vi "calcul.vi"(9 "In":dbl[](array[numeric]), 10 "Label (y)":dbl[](array[numeric]), 11 "Data (allx)":dbl[][](array[numeric])) -> (1 "PVAL":dbl[](array[numeric]), 3 "B":dbl[](array[numeric]))   [LabVIEW 2014]
uses:
  <vilib>/Analysis/Matrix/Datatypes/RealMatrix.ctl
  <vilib>/Analysis/baseanly.llb/Mean (DBL).vi
  <vilib>/Analysis/_algsub.llb/Real Vector Norm.vi
  <vilib>/Analysis/7linalg.llb/Real QR Decomposition.vi
  <vilib>/Analysis/baseanly.llb/Real A x B.vi
  <vilib>/Analysis/baseanly.llb/A x Vector.vi
  <vilib>/Analysis/baseanly.llb/Vector x A.vi
  <vilib>/Analysis/7linalg.llb/Create Special Real Matrix.vi
  <vilib>/Analysis/baseanly.llb/Real Inverse Matrix.vi
  <vilib>/Analysis/Matrix/Numeric/Subtract/Subtract - RM,RM.vi
  <vilib>/Analysis/Matrix/Numeric/Conversions/Matrix To Array - RM.vi
  <vilib>/Analysis/NI_AALPro.lvlib
  <vilib>/Analysis/NI_AALBase.lvlib
  <vilib>/Analysis/Matrix/NI_Matrix.lvlib
panel:
  out "SE":dbl[](array[numeric])
  out "s2":dbl[](array[numeric])
  out "df2":i32
  out "xr":dbl[][](array[numeric])
  out "Rrank":i16
  out "SSresid":dbl
  out "SStotal":dbl
  out "r":dbl[](array[numeric])
  out "sumxsq":dbl[](array[numeric])
  out "b2":dbl[](array[numeric])
  out "xx":dbl[](array[numeric])
  out "dfe":i32
  out "r2":T1
  out "N":i32
  out "yr":dbl[](array[numeric])
  out "se":dbl[](array[numeric])
  out "Rinv":T1
  out "rmse":dbl
  out "P":i32
  out "b":dbl[](array[numeric])
  out "Perm":i32[](array[numeric])
  out "R":T1
  out "Q":T1
  out "Large X":dbl[][](array[numeric])
  out "small x":dbl[][](array[numeric])
  out "nin":dbl
  out "tol":dbl
  # "Part1"
  # "Part3"
  # "INPUT DATA"
  # "Initialization of parameters"
  # "Part4"
  # "Part2"
  # "B_SE_maker"
  # "After comparison of (Rrank < nin)"
  # "get_PVAL"
  # "Calculation of SStotal, SSresid, dfe and etc"
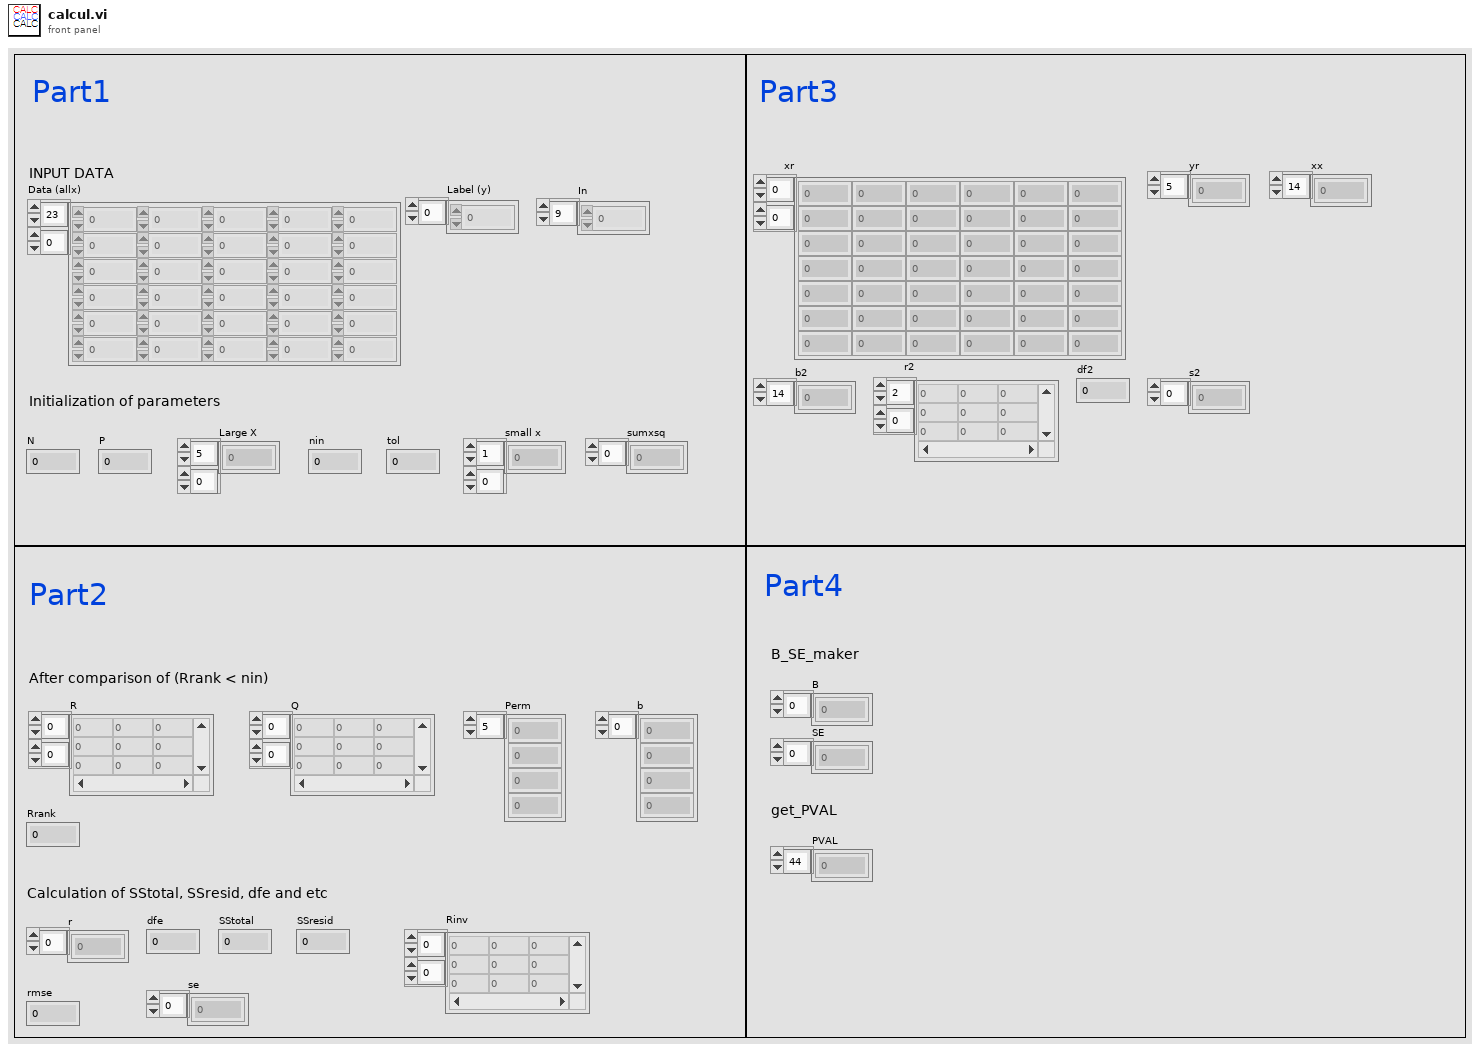
[diagram p1: front panel]
types:
  T1 = typedef "NI_Matrix.lvlib/RealMatrix.ctl" = dbl[][]
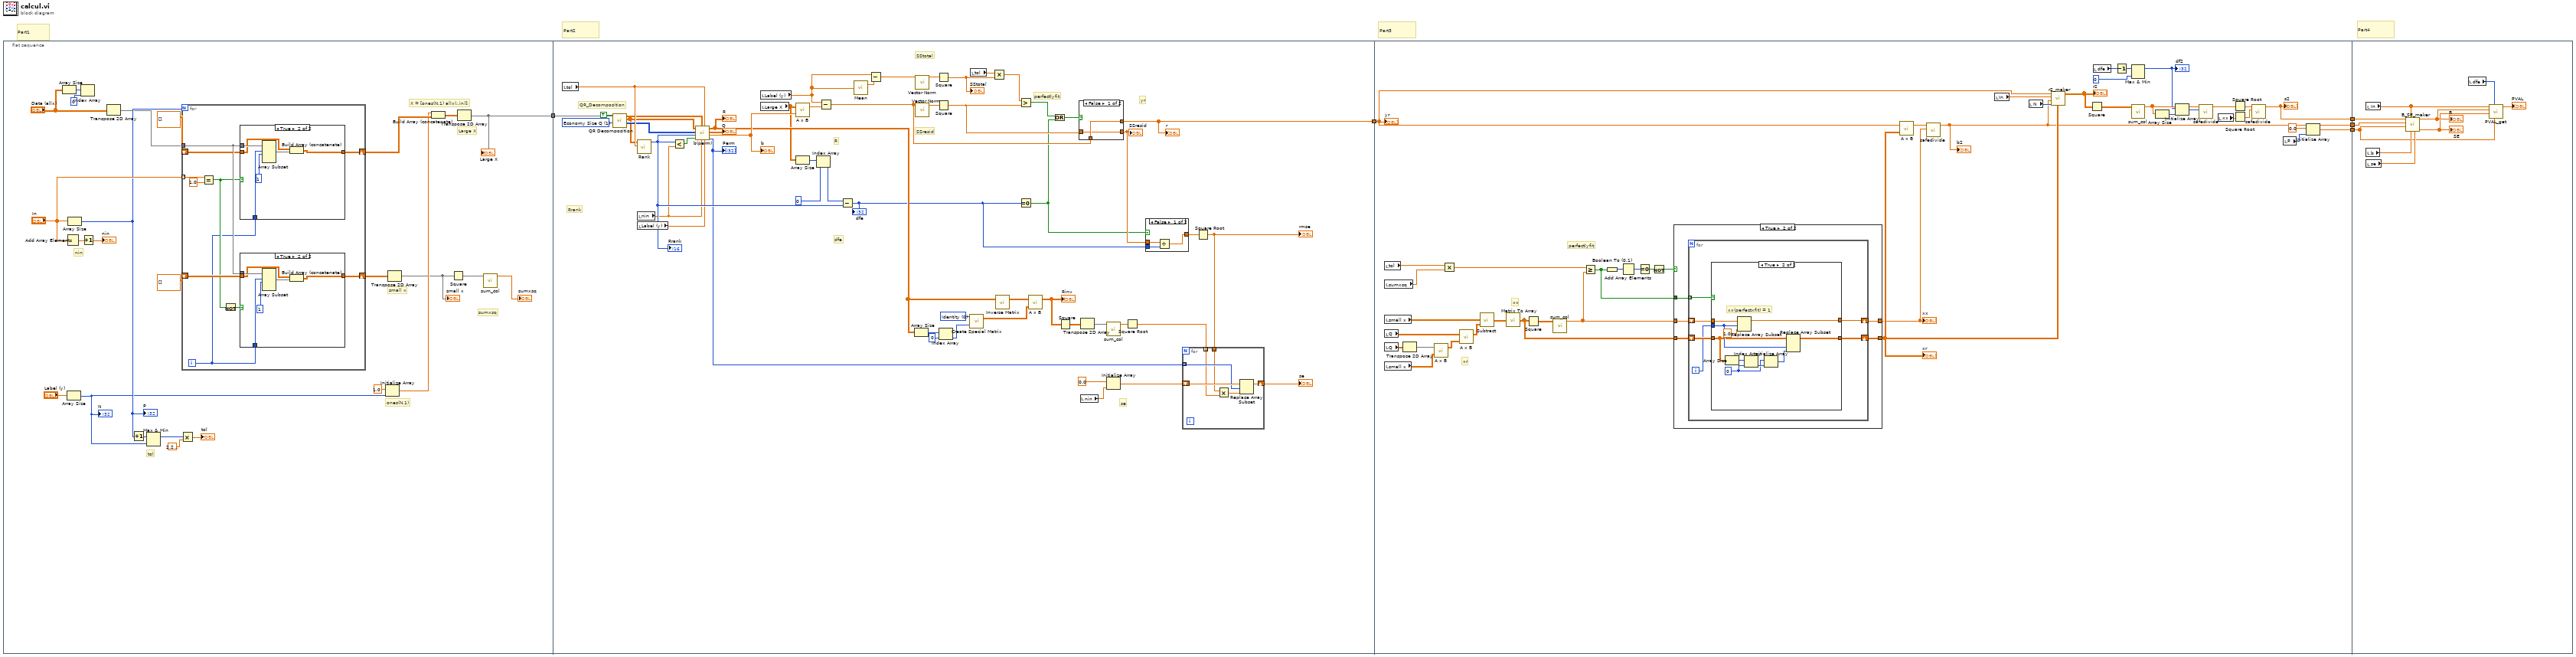
[diagram p0: block diagram]
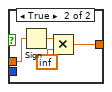
[diagram p4: hidden frame]
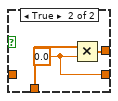
[diagram p5: hidden frame]
diagram:
  # "Part4"
  # "Part3"
  # "Part2"
  # "Part1"
  n1 = flat-sequence {
    tunnel: [w15] -> w5
    tunnel: w5 -> [w89]
    tunnel: [w59] -> w4
    tunnel: w4 -> [w148]
    tunnel: [w130] -> w3
    tunnel: [w152] -> w2
    tunnel: [w126] -> w1
    tunnel: w1 -> [w200]
    tunnel: w2 -> [w196]
    tunnel: w3 -> [w199]
    frame #0 {
      # "sumxsq"
      # "small x"
      # "Large X"
      # "tol"
      # "X = [ones(N,1) allx(:,in)];"
      # "ones(N,1)"
      # "nin"
      n2 = Array Size(array="Data (allx)") -> (size(s)=w25:i32[])
      n3 = Add Array Elements(numeric array="In") -> (sum=w29:dbl)
      n4 = Array Size(array="Label (y)") -> (size(s)=w8:i32)
      "N" <- w8
      n5 = Array Size(array="In") -> (size(s)=w21:i32)
      "P" <- w21
      n6 = Index Array(array=w25, index=0) -> ()  [unwired: 1 out]
      n7 = Increment(x=w29) -> (x+1=→"nin":dbl)
      n8 = Transpose 2D Array(2D array="Data (allx)") -> (transposed array=w6:dbl[][])
      n9 = Increment(x=w21) -> (x+1=w7:i32)
      n10 = Max & Min(x=w7, y=w8) -> (max(x,y)=w20:i32)  [unwired: 1 out]
      n11 = Multiply(x=w20, y=2.220446049250313e-16) -> (x*y=→"tol":dbl)
      n12 = for {
        N: w21 -> [_]
        tunnel: w6 -> [w37]
        tunnel: "In" -> [w40] mode=indexing
        shift-right: [w38] -> w23
        shift-left: dbl[][] [] -> [w36]
        shift-right: [w35] -> w17
        shift-left: dbl[][] [] -> [w34]
        i -> [w31]
        n13 = Equal?(x=w40, y=1.0) -> (x = y?=w32:bool)
        n14 = Not(x=w32) -> (.not. x?=w33:bool)
        n15 = case shown="True" w32 {
          tunnel: w37 -> [_ w54]
          tunnel: w31 -> [_ w49]
          tunnel: [w48 w51] -> w38
          tunnel: w36 -> [w48 w50]
          frame False {
          }
          frame True {
            n16 = Array Subset(array=w54, index (row)=w49, length (row)=1 ("length")) -> (w52:dbl[][])  [unwired: 2 in]
            n17 = Build Array (concatenate)(w50, w52) -> (w51:dbl[][])
          }
        }
        n18 = case shown="True" w33 {
          tunnel: w37 -> [_ w47]
          tunnel: w31 -> [_ w42]
          tunnel: [w41 w44] -> w35
          tunnel: w34 -> [w41 w43]
          frame False {
          }
          frame True {
            n19 = Array Subset(array=w47, index (row)=w42, length (row)=1 ("length")) -> (w45:dbl[][])  [unwired: 2 in]
            n20 = Build Array (concatenate)(w43, w45) -> (w44:dbl[][])
          }
        }
      }
      n21 = Initialize Array(1.0 ("element"), w8) -> (w13:dbl[])
      n22 = Transpose 2D Array(2D array=w17) -> (transposed array=w11:dbl[][])
      "small x" <- w11
      n23 = Build Array (concatenate)(w13, w23) -> (w22:dbl[][])
      n24 = Square(x=w11) -> (x^2=w10:dbl[][])
      n25 = Transpose 2D Array(2D array=w22) -> (transposed array=w15:dbl[][])
      "Large X" <- w15
      n26 = call "sum_col.vi"("Array"=w10) -> ("row_vec(sum)"=→"sumxsq":dbl[])  [unwired: 10 in]
    }
    frame #1 {
      w76 = 0 items=["Identity", "Diagonal", "Toeplitz", "Vandermonde", "Companion", "Hankel", "Hadamard", "Wilkinson", "Hilbert", "Inverse Hilbert", "Rosser", "Pascal"] ("matrix type")
      w90 = u16 1 items=["Full Size Q", "Economy Size Q", "No Q"] ("Q option")
      # "se"
      # "yr"
      # "perfectlyfit"
      # "SStotal"
      # "SSresid"
      # "dfe"
      # "R"
      # "Rrank"
      # "QR_Decomposition"
      n27 = local read "tol"() -> (w97:dbl)
      n28 = call-poly <vilib>:"QR Decomposition.vi"("Q option"=w90, "pivot?"=TRUE, "A"=w89) -> ("P"=w96:i32[][], "R"=w92:T1, "Q"=w93:T1)  [unwired: 5 in, 1 out]
      n29 = call "Rank.vi"("tol"=w97, "R"=w92) -> ("Numeric"=w100:i16)  [unwired: 9 in]
      "Rrank" <- w100
      n30 = local read "nin"() -> (w94:dbl)
      n31 = local read "Label (y)"() -> (w95:dbl[])
      n32 = Less?(x=w100, y=w94) -> (x < y?=w91:bool)
      n33 = call "b(perm).vi"("Label"=w95, "tol"=w97, "nin"=w94, "Q"=w93, "Boolean"=w91, "Rank"=w100, "P"=w96, "R"=w92) -> ("perm"=w60:i32[], "b(perm)"=w98:dbl[], "Q"=→"Q":T1, "R"=w75:T1)
      "R" <- w75
      "Perm" <- w60
      "b" <- w98
      n34 = local read "Label (y)"() -> (w102:dbl[])
      n35 = local read "Large X"() -> (w58:dbl[][])
      n36 = call-poly <vilib>:"A x B.vi"("Vector"=w98, "A"=w58) -> ("A x Vector"=w99:dbl[])  [unwired: 1 out]
      n37 = Array Size(array=w58) -> (size(s)=w57:i32[])
      n38 = Index Array(array=w57, index=0) -> (element=w55:i32)
      n39 = Subtract(x=w102, y=w99) -> (x-y=w77:dbl[])
      n40 = Subtract(x=w55, y=w100) -> (x-y=w64:i32)
      "dfe" <- w64
      n41 = call-poly <vilib>:"Mean.vi"("X"=w102) -> ("mean"=w101:dbl)  [unwired: 1 out]
      n42 = Subtract(x=w102, y=w101) -> (x-y=w78:dbl[])
      n43 = Array Size(array=w75) -> (size(s)=w74:i32[])
      n44 = call-poly <vilib>:"Vector Norm.vi"("Input Vector"=w78) -> ("norm"=w103:dbl)  [unwired: 9 in, 1 out]
      n45 = call-poly <vilib>:"Vector Norm.vi"("Input Vector"=w77) -> ("norm"=w104:dbl)  [unwired: 9 in, 1 out]
      n46 = Square(x=w103) -> (x^2=w66:dbl)
      "SStotal" <- w66
      n47 = Square(x=w104) -> (x^2=w63:dbl)
      n48 = Index Array(array=w74, index=0) -> (element=w72:i32)
      n49 = call-poly <vilib>:"Create Special Matrix.vi"("matrix type"=w76, "matrix size"=w72) -> ("Special Matrix"=w71:T1)  [unwired: 3 in, 1 out]
      n50 = local read "tol"() -> (w67:dbl)
      n51 = Multiply(x=w67, y=w66) -> (x*y=w65:dbl)
      n52 = call-poly <vilib>:"Inverse Matrix.vi"("Input Matrix"=w75) -> ("Inverse Matrix"=w87:T1)  [unwired: 1 in, 1 out]
      n53 = Greater?(x=w65, y=w63) -> (0:w105:bool)
      n54 = Equal To 0?(x=w64) -> (x = 0?=w61:bool)
      n55 = call-poly <vilib>:"A x B.vi"("B"=w71, "A"=w87) -> ("A x B"=w83:T1)  [unwired: 1 out]
      "Rinv" <- w83
      n56 = Or(x=w105, y=w61) -> (x .or. y?=w106:bool)
      n57 = Square(x=w83) -> (x^2=w70:T1)
      n58 = case shown="False" w106 {
        tunnel: w77 -> [w122 w125]
        tunnel: [w122 w124] -> w59
        tunnel: w63 -> [w121 _]
        tunnel: [w121 w123] -> w62
        frame False {
        }
        frame True {
          w123 = 0.0 ("y")
          n59 = Multiply(x=w125, y=w123) -> (x*y=w124:dbl[])
        }
      }
      "r" <- w59
      "SSresid" <- w62
      n60 = Transpose 2D Array(2D array=w70) -> (transposed array=w69:T1)
      n61 = local read "nin"() -> (w86:dbl)
      n62 = call "sum_col.vi"("Array"=w69) -> ("row_vec(sum)"=w68:dbl[])  [unwired: 10 in]
      n63 = Initialize Array(0.0 ("element"), w86) -> (w84:dbl[])
      n64 = Square Root(x=w68) -> (sqrt(x)=w81:dbl[])
      n65 = case shown="False" w61 {
        tunnel: [w114 w119] -> w88
        tunnel: w64 -> [w116 _]
        tunnel: w62 -> [w115 w118]
        frame False {
          n66 = Divide(x=w115, y=w116) -> (x/y=w114:dbl)
        }
        frame True {
          n67 = Sign(1:w118) -> (0:w120:dbl)
          n68 = Multiply(x=w120, y=inf) -> (x*y=w119:dbl)
        }
      }
      n69 = Square Root(x=w88) -> (sqrt(x)=w82:dbl)
      "rmse" <- w82
      n70 = for {
        tunnel: w60 -> [w112] mode=indexing
        shift-right: [w110] -> w80
        shift-left: w84 -> [w113]
        tunnel: w82 -> [w109]
        tunnel: w81 -> [w108] mode=indexing
        n71 = Multiply(x=w109, y=w108) -> (x*y=w111:dbl)
        n72 = Replace Array Subset(array=w113, new element=w111, index=w112) -> (w110:dbl[])
      }
      "se" <- w80
    }
    frame #2 {
      # "perfectlyfit"
      # "xx"
      # "xr"
      n73 = local read "tol"() -> (w161:dbl)
      n74 = local read "sumxsq"() -> (w133:dbl[])
      n75 = local read "small x"() -> (w163:dbl[][])
      n76 = local read "Q"() -> (w165:T1)
      n77 = local read "Q"() -> (w168:T1)
      n78 = local read "small x"() -> (w166:dbl[][])
      n79 = Transpose 2D Array(2D array=w168) -> (transposed array=w167:T1)
      n80 = call-poly <vilib>:"A x B.vi"("B"=w166, "A"=w167) -> ("A x B"=w164:T1)  [unwired: 1 out]
      n81 = Multiply(x=w161, y=w133) -> (x*y=w136:dbl[])
      n82 = call-poly <vilib>:"A x B.vi"("B"=w164, "A"=w165) -> ("A x B"=w162:T1)  [unwired: 1 out]
      n83 = call-poly <vilib>:"Subtract.vi"("Real Matrix B"=w162, "Real Matrix A"=w163) -> ("A - B"=w150:T1)
      n84 = call-poly <vilib>:"Matrix To Array.vi"("Real Matrix"=w150) -> ("Real 2D Array"=w134:dbl[][])
      n85 = Square(x=w134) -> (x^2=w138:dbl[][])
      n86 = call "sum_col.vi"("Array"=w138) -> ("row_vec(sum)"=w135:dbl[])  [unwired: 10 in]
      n87 = Greater Or Equal?(x=w136, y=w135) -> (x >= y?=w157:bool[])
      n88 = Boolean To (0,1)(Boolean=w157) -> (0, 1=w160:i16[])
      n89 = Add Array Elements(numeric array=w160) -> (sum=w159:i16)
      n90 = Equal To 0?(x=w159) -> (x = 0?=w158:bool)
      n91 = Not(x=w158) -> (.not. x?=w156:bool)
      n92 = case shown="True" w156 {
        tunnel: w157 -> [_ w175]
        tunnel: w135 -> [w170 w174]
        tunnel: w134 -> [w169 w173]
        tunnel: [w170 w172] -> w131
        tunnel: [w169 w171] -> w132
        frame False {
        }
        frame True {
          n93 = for {
            tunnel: w175 -> [w181] mode=indexing
            shift-right: [w179] -> w172
            shift-left: w174 -> [w180]
            shift-right: [w177] -> w171
            shift-left: w173 -> [w178]
            i -> [w176]
            n94 = case shown="True" w181 {
              tunnel: w180 -> [w183 w193]
              tunnel: w176 -> [_ w190]
              tunnel: [w183 w191] -> w179
              tunnel: w178 -> [w182 w188]
              tunnel: [w182 w189] -> w177
              frame False {
              }
              frame True {
                w184 = 0 ("index")
                # "xx(perfectxfit) = 1"
                n95 = Array Size(array=w188) -> (size(s)=w187:i32[])
                n96 = Replace Array Subset(array=w193, new element=1.0 ("new element/subarray"), index=w190) -> (w191:dbl[])
                n97 = Index Array(array=w187, index=w184) -> (element=w185:i32)
                n98 = Initialize Array(w184, w185) -> (w186:i32[])
                n99 = Replace Array Subset(array=w188, new element=w186, index (col)=w190) -> (w189:dbl[][])  [unwired: 1 in]
              }
            }
          }
        }
      }
      "xx" <- w131
      "xr" <- w132
      n100 = call-poly <vilib>:"A x B.vi"("Matrix A"=w132, "Vector V'"=w148) -> ("V' x A"=w155:dbl[])  [unwired: 1 out]
      n101 = call "safedivide.vi"("row_vec(sum)"=w131, "V' x A"=w155) -> ("Array"=w130:dbl[])  [unwired: 9 in]
      "b2" <- w130
      n102 = local read "In"() -> (w149:dbl[])
      n103 = local read "N"() -> (w151:i32)
      n104 = call "r2_maker.vi"("yr"=w148, "in"=w149, "b2"=w130, "N"=w151, "xr"=w132) -> ("r2"=w147:T1)  [unwired: 5 in]
      "r2" <- w147
      n105 = Square(x=w147) -> (x^2=w137:T1)
      n106 = local read "dfe"() -> (w143:i32)
      n107 = Decrement(x=w143) -> (x-1=w129:i32)
      n108 = Max & Min(x=w129, y=0 ("element")) -> (max(x,y)=w127:i32)  [unwired: 1 out]
      "df2" <- w127
      n109 = call "sum_col.vi"("Array"=w137) -> ("row_vec(sum)"=w146:dbl[])  [unwired: 10 in]
      n110 = Array Size(array=w146) -> (size(s)=w145:i32)
      n111 = Initialize Array(w127, w145) -> (w144:i32[])
      n112 = call "safedivide.vi"("row_vec(sum)"=w144, "V' x A"=w146) -> ("Array"=w142:dbl[])  [unwired: 9 in]
      n113 = local read "xx"() -> (w140:dbl[])
      n114 = Square Root(x=w142) -> (sqrt(x)=w141:dbl[])
      n115 = Square Root(x=w140) -> (sqrt(x)=w139:dbl[])
      n116 = call "safedivide.vi"("row_vec(sum)"=w139, "V' x A"=w141) -> ("Array"=w126:dbl[])  [unwired: 9 in]
      "s2" <- w126
      n117 = local read "P"() -> (w153:i32)
      n118 = Initialize Array(0.0 ("element"), w153) -> (w152:dbl[])
      "yr" <- w148
    }
    frame #3 {
      n119 = local read "In"() -> (w203:dbl[])
      n120 = local read "b"() -> (w198:dbl[])
      n121 = local read "se"() -> (w197:dbl[])
      n122 = call "B_SE_maker.vi"("se"=w197, "b"=w198, "In"=w203, "zeros(P,1)\nB/SE"=w196, "b2"=w199, "s2"=w200) -> ("SE"=w194:dbl[], "B"=w195:dbl[])  [unwired: 4 in]
      "B" <- w195
      "SE" <- w194
      n123 = local read "dfe"() -> (w201:i32)
      n124 = call "PVAL_get.vi"("zeros(P,1)"=w196, "dfe"=w201, "SE"=w194, "B"=w195, "In"=w203) -> ("PVAL"=→"PVAL":dbl[])  [unwired: 6 in]
    }
  }
